vi "Multirecord Acquisition (FPGA) - original.vi"() -> ()   [LabVIEW 2021]
doc: "Use this VI as a template for the reconfigurable oscilloscope acquisition design. The block diagram is divided into three main loops.\n\nRegister Bus: This loop initializes the registers that are needed to support the configuration of the device. The FIFO bus, on the left, allows all the other design libraries to communicate with one another. This loop is very important to support the proper behavior of the instrument design library components.\n\nAcquisition: Acquires data from the I/O channels and writes the data into the record memory using the <B>Write</B> VI of the Multirecord Acquisition instrument design library. This VI also evaluates the various acquisition triggers and decides whether to acquire each data value in record memory. The host level VI (Fetch Record.vi) can read acquired records from the DRAM. The data is stored in 2 DRAM banks, each with 768 MB of storage.\n\nFetch: The recorded data is retrieved when the <B>Fetch Single Record</B> VI is run from the host VI. The <B>Write to Fetch DMA FIFO</B> VI writes data to the acq.fetch fifo 0 to transmit record data form the FPGA to the record fetch VIs on the host. This DMA FIFO must have a predefined name based on the instance parameter. By default, it is 0 (since the associated terminal on the <B>Create Resources DRAM Write Read</B> VI is unwired), so the connected FIFO is named acq.fetch fifo 0."
uses:
  Trigger/SubVIs/Types/Trigger Type.ctl
  <instrlib>/_niInstr/Data Trigger/v1/Shared/Public/Level Configuration FXP(+-,18,1).ctl
  <instrlib>/_niInstr/Data Trigger/v1/Shared/Public/Level Configuration Trigger When.ctl
  <instrlib>/_niInstr/Data Trigger/v1/Shared/Public/Edge Configuration FXP(+-,18,1).ctl
  <instrlib>/_niInstr/Data Trigger/v1/Shared/Public/Edge Configuration Trigger Slope.ctl
  FPGA Interface Typedefinitions/Trigger Combination Type.ctl
  <vilib>/Platform/TimedLoop/XDataNode/timing_clust.ctl
  <vilib>/Platform/TimedLoop/XDataNode/nitl_modes.ctl
  <vilib>/Platform/TimedLoop/XDataNode/wakeup.ctl
  <instrlib>/_niInstr/FIFO Register Bus/v1/FPGA/niInstr FIFO Register Bus v1 FPGA.lvclass
  C:/Program Files (x86)/National Instruments/LabVIEW 2021/instr.lib/_niInstr/Instruction Framework/v1/FPGA/Interfaces/Instruction Producer/Instruction Producer.lvclass
  <instrlib>/_niInstr/Multirecord Acquisition/Common/v1/FPGA/niInstr Multirecord Acquisition Common v1 FPGA.lvclass
  C:/Program Files (x86)/National Instruments/LabVIEW 2021/instr.lib/_niInstr/Multirecord Acquisition/Interface/v1/FPGA/niInstr Multirecord Acquisition v1 FPGA.lvclass
  <vilib>/rvi/Emulation/niFpgaSctlEmulationGetInTimedLoop.vi
  <vilib>/rvi/Emulation/niFpgaEmulationReportErrorSimple.vi
  <vilib>/rvi/Emulation/niFpgaGetClockAttributes.vi
  <vilib>/rvi/Emulation/niFpgaCriticalErrorInLSC.vi
  <instrlib>/_niInstr/Multirecord Acquisition/Common/v1/FPGA/Private/Create Fetch DMA FIFO Resources U8x32.vi
  <instrlib>/_niInstr/Multirecord Acquisition/Common/v1/FPGA/Private/Create Resources DRAM U384x2 U768 Write Read.vi
  <instrlib>/_niInstr/Multirecord Acquisition/Interface/v1/FPGA/Private/Retrieve Record U16 Wrapper.vi
  <instrlib>/_niInstr/Multirecord Acquisition/Interface/v1/FPGA/Private/Write to Fetch DMA FIFO U16 Wrapper.vi
  <vilib>/rvi/eio/common/nirviEmuTemplateMethod_errors.vi
  <instrlib>/HSAI-RIO/Config/Group A/v1/FPGA/Digital Correction/Validate 8 Channel Data.vi
  <instrlib>/HSAI-RIO/Config/Group A/v1/FPGA/Digital Correction/Digital Correction (8 Ch).vi
  <instrlib>/HSAI-RIO/Config/Group A/v1/FPGA/Digital Correction/FIR Filter (8 Ch).vi
  DSP/SubVIs/Integer decimationx8ch.vi
  Data Type Conversion/SubVIs/Remove Overflow FXP(+-,18,1)x8ch.vi
  <instrlib>/_niInstr/Channel/v1/FPGA/Private/Select/Select FXP(+-,18,1,)xNspcx8ch.vi
  Data Type Conversion/SubVIs/Data Type Conversion FXP(+-,18,1) to I16x8ch.vi
  <instrlib>/_niInstr/Channel/v1/FPGA/Private/Select and Interleave/Select And Interleave I16xNspcx8ch.vi
  Trigger/Trigger FXP(+,-,18,1).vi
  <instrlib>/_niInstr/Multirecord Acquisition/Interface/v1/FPGA/Private/Write I16 Wrapper.vi
  <vilib>/Platform/TimedLoop/XDataNode/XDataNode.xnode
  <vilib>/eio/EIONode/EIONode.xnode
  <instrlib>/_niInstr/Instruction Framework/v1/FPGA/Top Level Bus/Register Configuration/Register Configuration.lvclass
  <vilib>/Platform/TimedLoop/XDataNode/XDNodeRunTimeDep.lvlib
  <instrlib>/_niInstr/Multirecord Acquisition/Interface/v1/FPGA/niInstr Multirecord Acquisition v1 FPGA.lvclass
  <vilib>/rvi/LocalResourceManager/LocalResourceManager.xnode
  <vilib>/rvi/eio/common/nirviEmuReportErrorAndStop.vi
  <vilib>/rvi/DataTransferAndStorage/Container/Common/niFpgaContainerGetUniqueNameForEmu.vi
  <vilib>/rvi/DataTransferAndStorage/Container/Common/niFpgaContainerSetEmuInfo.vi
  <instrlib>/_niInstr/Channel/v1/FPGA/niInstr Channel v1 FPGA.lvlib
  <instrlib>/_niInstr/Basic Elements/v1/FPGA/niInstr Basic Elements v1 FPGA.lvlib
  <instrlib>/HSAI-RIO/Config/Group A/v1/FPGA/Digital Correction/Digital Correction.lvclass
  <instrlib>/HSAI-RIO/Config/Group A/v1/FPGA/Config Registers/Config Registers.lvclass
  <instrlib>/_niInstr/Data Trigger/v1/Shared/niInstr Data Trigger v1 Shared.lvlib
  <instrlib>/_niInstr/Multirecord Acquisition/Common/v1/FPGA/Private/Create Resources DRAM U384.vi
  <instrlib>/_niInstr/Multirecord Acquisition/Common/v1/FPGA/Private/Create Resources BRAM U384.vi
  Emulation/SubVIs/2 Element Generate Sine Cos Data FXP(+,-,14,1).vi
  <instrlib>/HSAI-RIO/Config/Group A/v1/FPGA/Digital Correction/Validate 4 Channel Data.vi
  <instrlib>/HSAI-RIO/Config/Group A/v1/FPGA/Digital Correction/Digital Correction (4 Ch).vi
  <instrlib>/_niInstr/Channel/v1/FPGA/Private/Select/Select FXP(+-,18,1,)xNspcx4ch.vi
  C:/Program Files (x86)/National Instruments/LabVIEW 2021/instr.lib/_niInstr/Multirecord Acquisition/Common/v1/FPGA/niInstr Multirecord Acquisition Common v1 FPGA.lvclass
  Data Type Conversion/SubVIs/Remove Overflow FXP(+-,18,1)x4ch.vi
  Data Type Conversion/SubVIs/Data Type Conversion FXP(+-,18,1) to I16x4ch.vi
  <instrlib>/_niInstr/Channel/v1/FPGA/Private/Select and Interleave/Select And Interleave I16xNspcx4ch.vi
  DSP/SubVIs/Integer decimationx4ch.vi
  <instrlib>/HSAI-RIO/Config/Group A/v1/FPGA/Digital Correction/FIR Filter (4 Ch).vi
  <instrlib>/_niInstr/Multirecord Acquisition/Common/v1/FPGA/Private/Create Resources BRAM U768.vi
  FPGA Interface Typedefinitions/FPGA Interface Typedefinitions.lvlib
panel:
  in  "trigger.rearm delay":u16=2
  in  "start trigger":bool=TRUE
  in  "trigger.type B":T1
  in  "reset":bool
  in  "trigger.combination type":T2
  in  "trigger.edge B":T3
  in  "trigger.level B":T5
  in  "trigger.edge A":T3
  in  "trigger.level A":T5
  in  "trigger.type A":T1
  in  "trigger.channel A":u8
  in  "trigger.channel B":u8
  out "fifo reg bus data 0":u64
  out "fifo reg bus status 0":u32
  in  "fifo reg bus ctrl 0":u32
  out "overflow":bool
  in  "dsp.decimation factor":u16
  out "overload":bool
  in  "channel.enable mask":u16=65535 format="%.0b"
  in  "channel.number of channels":u8=8
  # "Register Bus Controls"
  # "FPGA"
  # "Acquisition Loop Controls"
  # "DSP"
  # "Trigger"
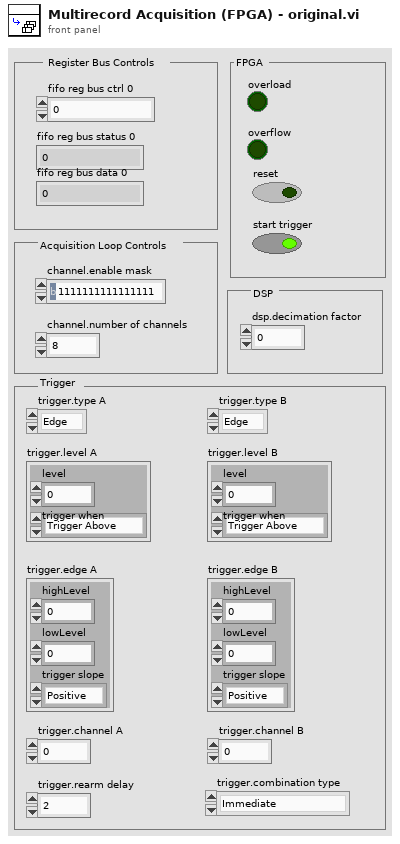
[diagram p1: front panel]
types:
  T1 = typedef "Trigger Type.ctl" = enum16{"Edge", "Level", "Custom"}
  T2 = typedef "FPGA Interface Typedefinitions.lvlib/Trigger Combination Type.ctl" = enum16{"Immediate", "A", "B", "OR", "AND", "A THEN B", "B THEN A", "High Resolution"}
  T3 = typedef "niInstr Data Trigger v1 Shared.lvlib/Edge Configuration FXP(+-,18,1).ctl" = cluster{"highLevel":fxp<+/-,18,1>, "lowLevel":fxp<+/-,18,1>, "trigger slope":T4}
  T4 = typedef "niInstr Data Trigger v1 Shared.lvlib/Edge Configuration Trigger Slope.ctl" = enum8{"Positive", "Negative"}
  T5 = typedef "niInstr Data Trigger v1 Shared.lvlib/Level Configuration FXP(+-,18,1).ctl" = cluster{"level":fxp<+/-,18,1>, "trigger when":T6}
  T6 = typedef "niInstr Data Trigger v1 Shared.lvlib/Level Configuration Trigger When.ctl" = enum8{"Trigger Above", "Trigger Below"}
  T7 = cluster{"memory 1":refnum<k21>, "memory 2":refnum<k21>}
  T8 = typedef "XDNodeRunTimeDep.lvlib/timing_clust.ctl" = cluster{"Expected End [f-1]":u64, "Actual End [f-1]":u64, "Finished Late? [f-1]":bool, "Expected End [i-1]":u64, "Actual End [i-1]":u64, "Finished Late? [i-1]":bool, "Expected Start [i]":u64, "Actual Start [i]":u64, "Expected Start [f]":u64, "Actual Start [f]":u64, "Source Name":string, "Structure Name":string, "Period":i64, "Deadline":i64, "Offset":i64, "Start":i64, "Priority":i32, "Timeout":i32, "Mode":T9, "Wakeup Reason":T10, "Error":errorcluster, "Source Type":string, "Secondary Source Type":string, "Global End Time":u64, "Global Start Time":u64, "Frame Duration":u64, "Iteration Duration":u64, "Assigned CPU":i32, "I/O Scan Engine Mode":u32}
  T9 = typedef "XDNodeRunTimeDep.lvlib/nitl_modes.ctl" = enum32{"No Change", "Process missed periods, maintain original phase", "Discard missed periods, maintain original phase", "Process missed periods, ignore original phase", "Discard missed periods, ignore original phase"}
  T10 = typedef "XDNodeRunTimeDep.lvlib/wakeup.ctl" = enum32{"Normal", "Aborted", "Asynchronous wakeup", "Timing source error", "Timed loop error", "Timeout"}
  T11 = typedef "niInstr Multirecord Acquisition v1 FPGA.lvclass/Timestamp.ctl" = cluster{"timestamp":u64, "valid":bool}
  T12 = typedef "niInstr Types v1 Shared.lvlib/Input Triggers.ctl" = cluster{"start":bool, "advance":bool, "reference":bool, "start trigger index":u16, "advance trigger index":u16, "reference trigger index":u16, "reference trigger correction cycle count":u32}
  T13 = cluster{"Channel 0":fxp<+/-,14,1>[], "Channel 1":fxp<+/-,14,1>[], "Channel 2":fxp<+/-,14,1>[], "Channel 3":fxp<+/-,14,1>[], "Channel 4":fxp<+/-,14,1>[], "Channel 5":fxp<+/-,14,1>[], "Channel 6":fxp<+/-,14,1>[], "Channel 7":fxp<+/-,14,1>[]}
  T14 = cluster{"Channel 0":fxp<+/-,18,1>[], "Channel 1":fxp<+/-,18,1>[], "Channel 2":fxp<+/-,18,1>[], "Channel 3":fxp<+/-,18,1>[], "Channel 4":fxp<+/-,18,1>[], "Channel 5":fxp<+/-,18,1>[], "Channel 6":fxp<+/-,18,1>[], "Channel 7":fxp<+/-,18,1>[]}
  T15 = cluster{"channel 0":fxp<+/-,18,1>[], "channel 1":fxp<+/-,18,1>[], "channel 2":fxp<+/-,18,1>[], "channel 3":fxp<+/-,18,1>[], "channel 4":fxp<+/-,18,1>[], "channel 5":fxp<+/-,18,1>[], "channel 6":fxp<+/-,18,1>[], "channel 7":fxp<+/-,18,1>[]}
  T16 = cluster{"channel 0":i16[], "channel 1":i16[], "channel 2":i16[], "channel 3":i16[], "channel 4":i16[], "channel 5":i16[], "channel 6":i16[], "channel 7":i16[]}
  T17 = typedef "niInstr Types v1 Shared.lvlib/Sample Format.ctl" = cluster{"bits per channel":u16, "samples per clock":u16, "channels":u8}
  T18 = cluster{"Channel 0":fxp<+/-,14,1>[], "Channel 1":fxp<+/-,14,1>[], "Channel 2":fxp<+/-,14,1>[], "Channel 3":fxp<+/-,14,1>[]}
  T19 = cluster{"Channel 0":fxp<+/-,18,1>[], "Channel 1":fxp<+/-,18,1>[], "Channel 2":fxp<+/-,18,1>[], "Channel 3":fxp<+/-,18,1>[]}
  T20 = cluster{"channel 0":fxp<+/-,18,1>[], "channel 1":fxp<+/-,18,1>[], "channel 2":fxp<+/-,18,1>[], "channel 3":fxp<+/-,18,1>[]}
  T21 = cluster{"channel 0":i16[], "channel 1":i16[], "channel 2":i16[], "channel 3":i16[]}
  T22 = typedef "niInstr Multirecord Acquisition v1 FPGA.lvclass/Events.ctl" = cluster{"ready for start":bool, "ready for advance":bool, "ready for reference":bool, "end of record":bool, "done":bool, "start trigger":bool, "advance trigger":bool, "reference trigger":bool, "start trigger index":u16, "advance trigger index":u16, "reference trigger index":u16}
  T23 = typedef "niInstr Multirecord Acquisition v1 FPGA.lvclass/Retrieve Data Info.ctl" = cluster{"read request size (bits)":u64, "valid data offset (bits)":u16, "valid data size (bits)":u16, "first sample of request":bool, "last sample of request":bool, "Token":T24}
  T24 = typedef "niInstr Types v1 Shared.lvlib/Token.ctl" = cluster{"identifier":u8, "value":u32}
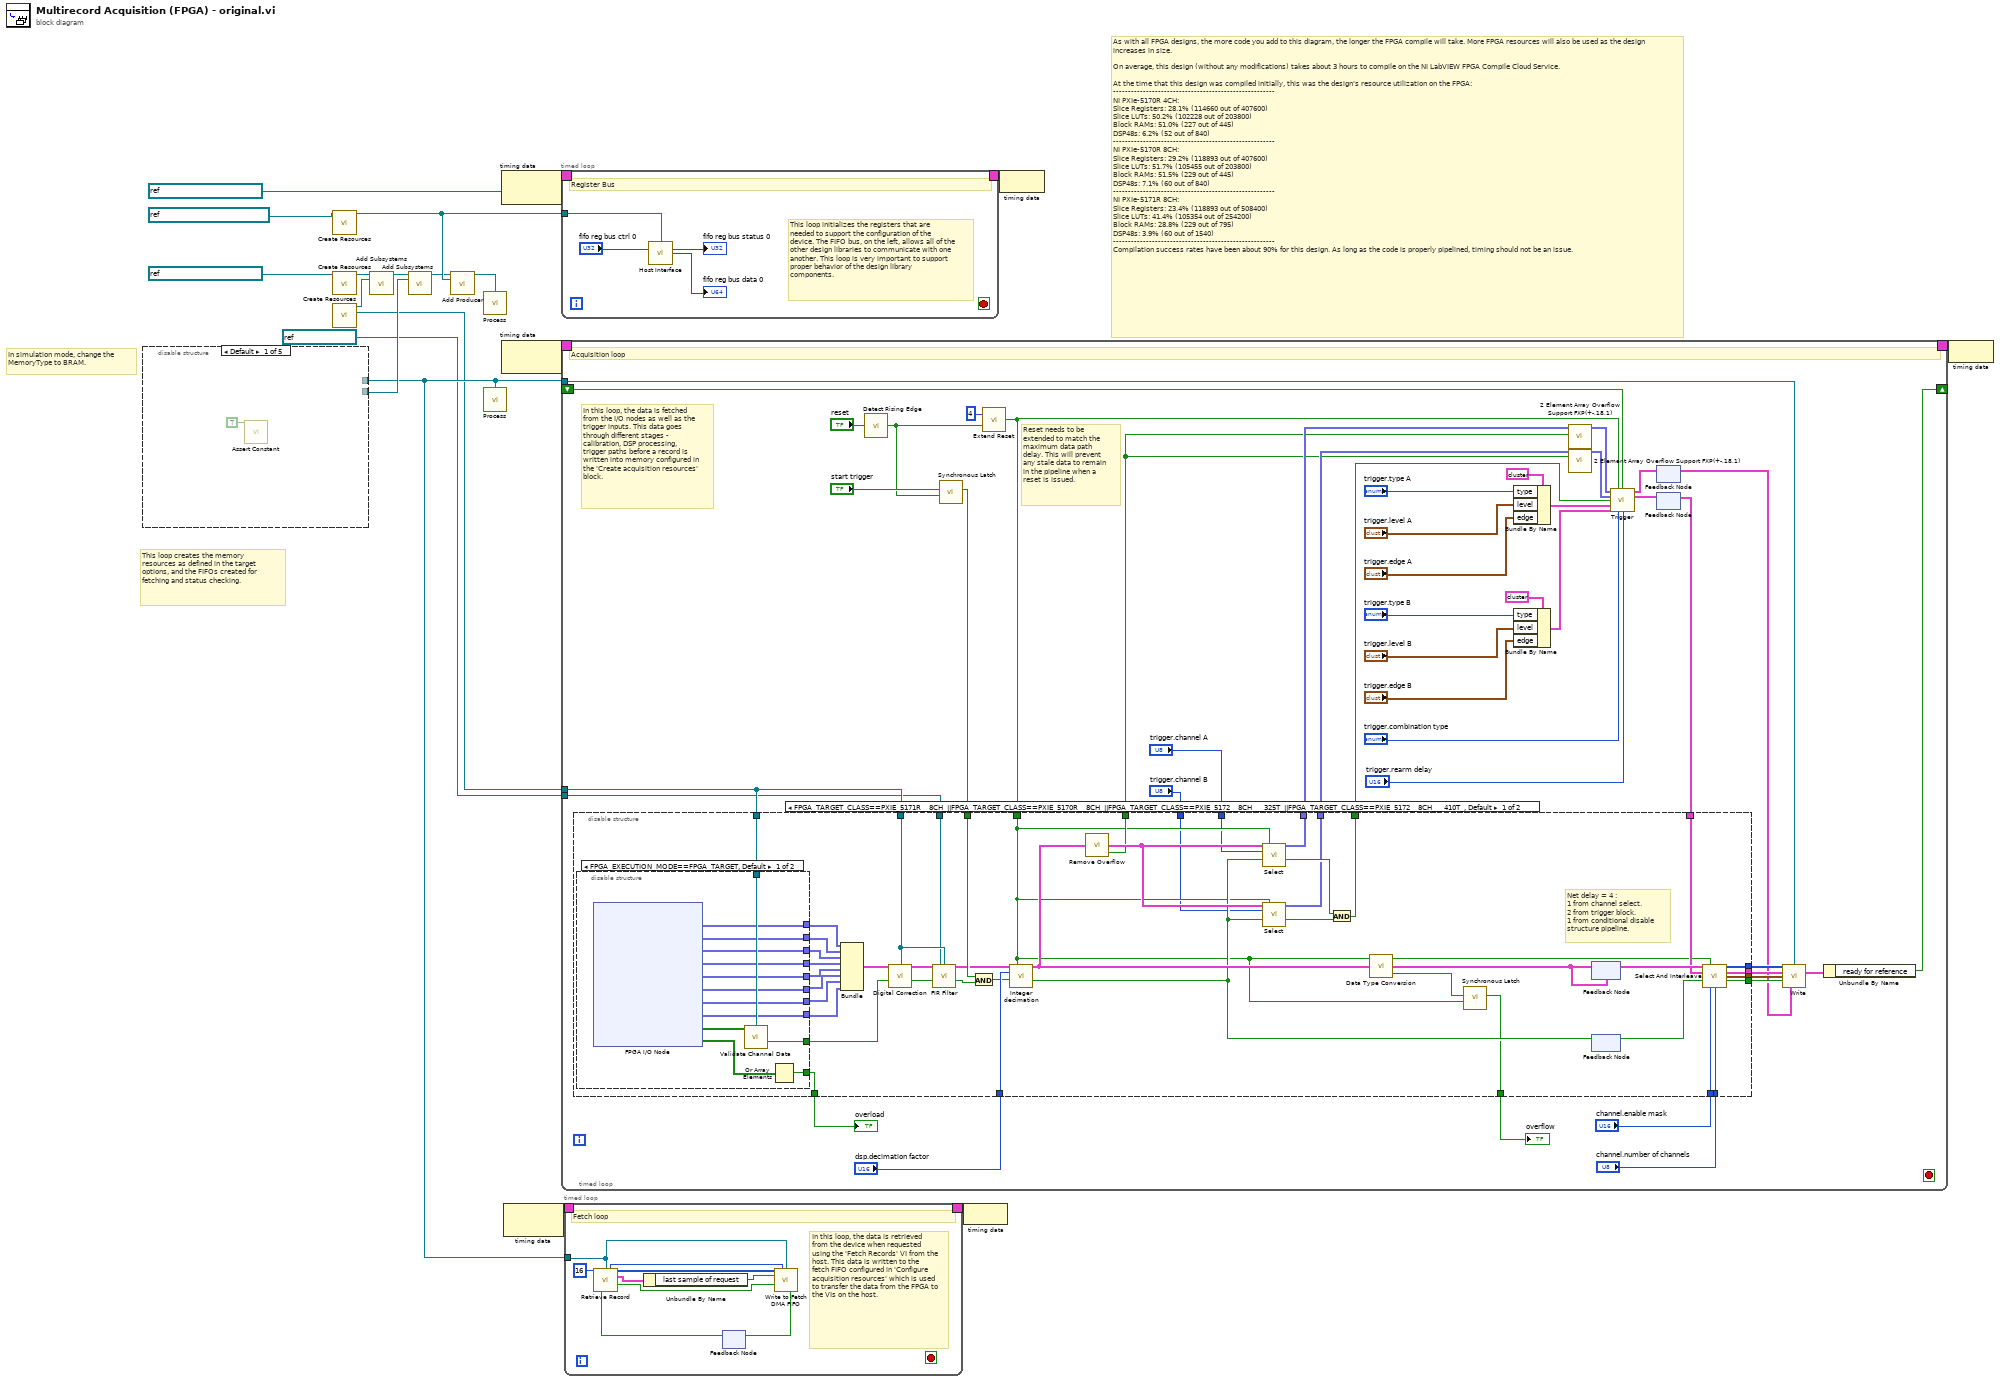
[diagram p0: block diagram]
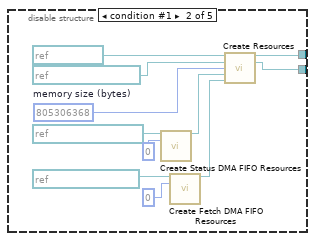
[diagram p2: hidden frame]
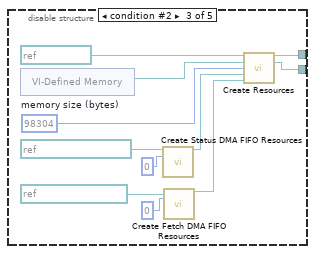
[diagram p3: hidden frame]
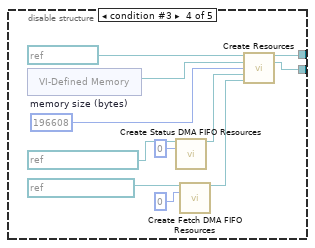
[diagram p4: hidden frame]
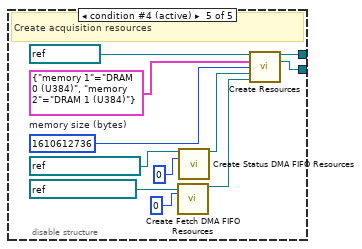
[diagram p5: hidden frame]
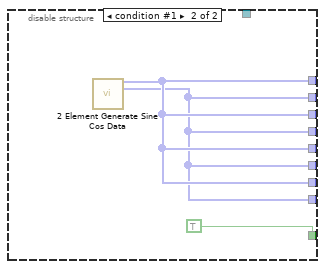
[diagram p6: hidden frame]
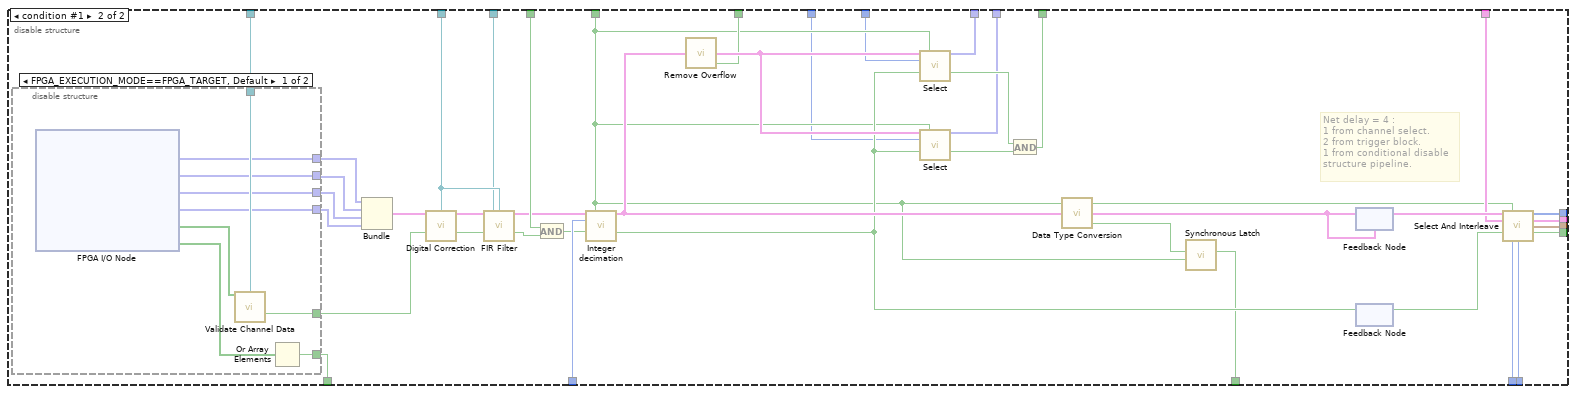
[diagram p7: hidden frame]
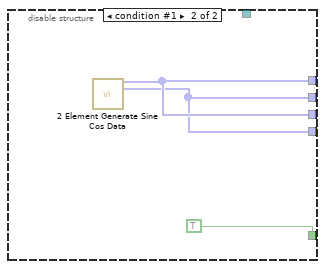
[diagram p8: hidden frame]
diagram:
  # "In simulation mode, change the MemoryType to BRAM."
  # "This loop creates the memory resources as defined in the target options, and the FIFOs created for fetching and status checking."
  # "As with all FPGA designs, the more code you add to this diagram, the longer the FPGA compile will take. More FPGA resources will also be used as the design increases in size.\n\nOn average, this design (without any modifications) takes about 3 hours to compile on the NI LabVIEW FPGA Compile Cloud Service. \n\nAt the time that this design was compiled initially, this was the design's resource utilization on the FPGA:\n------------------------------------------------------\nNI PXIe-5170R 4CH:\nSlice Registers: 28.1% (114660 out of 407600)\nSlice LUTs: 50.2% (102228 out of 203800)\nBlock RAMs: 51.0% (227 out of 445)\nDSP48s: 6.2% (52 out of 840)\n------------------------------------------------------\nNI PXIe-5170R 8CH:\nSlice Registers: 29.2% (118893 out of 407600)\nSlice LUTs: 51.7% (105455 out of 203800)\nBlock RAMs: 51.5% (229 out of 445)\nDSP48s: 7.1% (60 out of 840)\n------------------------------------------------------\nNI PXIe-5171R 8CH:\nSlice Registers: 23.4% (118893 out of 508400)\nSlice LUTs: 41.4% (105354 out of 254200)\nBlock RAMs: 28.8% (229 out of 795)\nDSP48s: 3.9% (60 out of 1540)\n------------------------------------------------------\nCompilation success rates have been about 90% for this design. As long as the code is properly pipelined, timing should not be an issue."
  n1 = disable-structure shown="Default" {
    disable-tunnel: [_ w29 w40 w51 w62] -> w4
    disable-tunnel: [_ w26 w36 w47 w59] -> w7
    frame condition #0 {
      n2 = call <instrlib>:"Assert Constant.vi"("constant terminal"=TRUE) -> ()  [unwired: 15 in]
    }
    frame condition #1 {
      w30 = u64 805306368  # memory size (bytes)
      n3 = call <instrlib>:"Create Status DMA FIFO Resources.vi"("status dma fifo in"=refnum<k21> "acq.status fifo 0" ("status dma fifo"), "fifo instance"=u8 0) -> ("status dma fifo out"=w21:refnum<class "niInstr Status FIFO v1 FPGA.lvclass">)  [unwired: 13 in]
      n4 = call-poly <instrlib>:"Create Fetch DMA FIFO Resources.vi"("fetch dma fifo in"=refnum<k21> "acq.fetch fifo 0", "fifo instance"=u8 0) -> ("fetch dma fifo out"=w27:refnum<class "niInstr Fetch FIFO v1 FPGA.lvclass">)  [unwired: 13 in]
      n5 = call-poly <instrlib>:"Create Resources.vi"("memory clock"=refnum<k21> "160MHz" ("process clock"), "memory"=refnum<k21> "DRAM 0 (U384)" ("dram"), "memory size (bytes)"=w30, "status dma fifo resources"=w21, "fetch dma fifo resources"=w27) -> ("acquisition resources"=w29:refnum<class "niInstr Multirecord Acquisition Common v1 FPGA.lvclass">, "acquisition subsystem"=w26:refnum<class "Address Space Collection.lvclass">)  [unwired: 9 in]
    }
    frame condition #2 {
      w41 = u64 98304  # memory size (bytes)
      n6 = xnode "VI-Defined Memory"() -> ("Memory Out"=w42:refnum<k21>)
      n7 = call <instrlib>:"Create Status DMA FIFO Resources.vi"("status dma fifo in"=refnum<k21> "acq.status fifo 0" ("status dma fifo"), "fifo instance"=u8 0) -> ("status dma fifo out"=w33:refnum<class "niInstr Status FIFO v1 FPGA.lvclass">)  [unwired: 13 in]
      n8 = call-poly <instrlib>:"Create Fetch DMA FIFO Resources.vi"("fetch dma fifo in"=refnum<k21> "acq.fetch fifo 0", "fifo instance"=u8 0) -> ("fetch dma fifo out"=w37:refnum<class "niInstr Fetch FIFO v1 FPGA.lvclass">)  [unwired: 13 in]
      n9 = call-poly <instrlib>:"Create Resources.vi"("memory clock"=refnum<k21> "160MHz" ("process clock"), "memory"=w42, "memory size (bytes)"=w41, "status dma fifo resources"=w33, "fetch dma fifo resources"=w37) -> ("acquisition resources"=w40:refnum<class "niInstr Multirecord Acquisition Common v1 FPGA.lvclass">, "acquisition subsystem"=w36:refnum<class "Address Space Collection.lvclass">)  [unwired: 9 in]
    }
    frame condition #3 {
      w52 = u64 196608  # memory size (bytes)
      n10 = xnode "VI-Defined Memory"() -> ("Memory Out"=w53:refnum<k21>)
      n11 = call <instrlib>:"Create Status DMA FIFO Resources.vi"("status dma fifo in"=refnum<k21> "acq.status fifo 0" ("status dma fifo"), "fifo instance"=u8 0) -> ("status dma fifo out"=w45:refnum<class "niInstr Status FIFO v1 FPGA.lvclass">)  [unwired: 13 in]
      n12 = call-poly <instrlib>:"Create Fetch DMA FIFO Resources.vi"("fetch dma fifo in"=refnum<k21> "acq.fetch fifo 0", "fifo instance"=u8 0) -> ("fetch dma fifo out"=w48:refnum<class "niInstr Fetch FIFO v1 FPGA.lvclass">)  [unwired: 13 in]
      n13 = call-poly <instrlib>:"Create Resources.vi"("memory clock"=refnum<k21> "160MHz" ("process clock"), "memory"=w53, "memory size (bytes)"=w52, "status dma fifo resources"=w45, "fetch dma fifo resources"=w48) -> ("acquisition resources"=w51:refnum<class "niInstr Multirecord Acquisition Common v1 FPGA.lvclass">, "acquisition subsystem"=w47:refnum<class "Address Space Collection.lvclass">)  [unwired: 9 in]
    }
    frame condition #4 (active) {
      w64 = u64 1610612736  # memory size (bytes)
      # "Create acquisition resources"
      n14 = call-poly <instrlib>:"Create Fetch DMA FIFO Resources.vi"("fetch dma fifo in"=refnum<k21> "acq.fetch fifo 0", "fifo instance"=u8 0) -> ("fetch dma fifo out"=w61:refnum<class "niInstr Fetch FIFO v1 FPGA.lvclass">)  [unwired: 13 in]
      n15 = call <instrlib>:"Create Status DMA FIFO Resources.vi"("status dma fifo in"=refnum<k21> "acq.status fifo 0" ("status dma fifo"), "fifo instance"=u8 0) -> ("status dma fifo out"=w56:refnum<class "niInstr Status FIFO v1 FPGA.lvclass">)  [unwired: 13 in]
      n16 = call-poly <instrlib>:"Create Resources.vi"("memory clock"=refnum<k21> "160MHz" ("process clock"), "memory"=T7 {"memory 1"="DRAM 0 (U384)", "memory 2"="DRAM 1 (U384)"}, "memory size (bytes)"=w64, "status dma fifo resources"=w56, "fetch dma fifo resources"=w61) -> ("acquisition resources"=w62:refnum<class "niInstr Multirecord Acquisition Common v1 FPGA.lvclass">, "acquisition subsystem"=w59:refnum<class "Address Space Collection.lvclass">)  [unwired: 9 in]
    }
  }
  n17 = call <instrlib>:"Create Resources.vi"("instruction fifo"=refnum<k21> "reg.host instruction fifo 0" ("FIFO")) -> ("fifo register bus"=w6:refnum<class "niInstr FIFO Register Bus v1 FPGA.lvclass">)  [unwired: 14 in]
  n18 = call <instrlib>:"Create Resources.vi"("register clock"=refnum<k21> "40 MHz Onboard Clock" ("Source Name")) -> ("register configuration"=w10:refnum<class "Register Configuration.lvclass">)  [unwired: 14 in]
  n19 = call <instrlib>:"Create Resources.vi"() -> ("config subsystems"=w8:refnum<class "Address Space Collection.lvclass">, "digital correction resources"=w1:refnum<class "Digital Correction.lvclass">)  [unwired: 14 in]
  n20 = call-dynamic "Add Subsystems.vi"("register configuration in"=w10, "subsystems"=w8) -> ("register configuration out"=w9:refnum<class "Register Configuration.lvclass">)  [unwired: 13 in]
  n21 = call-dynamic "Add Subsystems.vi"("register configuration in"=w9, "subsystems"=w7) -> ("register configuration out"=w3:refnum<class "Register Configuration.lvclass">)  [unwired: 13 in]
  n22 = call-dynamic "Add Producer.vi"("register configuration in"=w3, "instruction producer"=w6) -> ("register configuration out"=w5:refnum<class "Register Configuration.lvclass">)  [unwired: 13 in]
  n23 = call-dynamic "Process.vi"("register configuration"=w5) -> ()  [unwired: 15 in]
  n24 = call-dynamic "Process.vi"("acquisition resources"=w4) -> ()  [unwired: 15 in]
  n25 = node-c288(refnum<k21> "40 MHz Onboard Clock" ("Source Name")) -> (w19:T8)
  n26 = node-c288() -> (w17:T8)  [unwired: 1 in]
  n27 = node-c288() -> (w15:T8)  [unwired: 1 in]
  n28 = timed-loop {
    timing: w19 -> [_]
    timing-out: [_] -> w18
    tunnel: w6 -> [w68]
    stop <- _ stop-if-true
    # "This loop initializes the registers that are needed to support the configuration of the device. The FIFO bus, on the left, allows all of the other design libraries to communicate with one another. This loop is very important to support proper behavior of the design library components."
    # "Register Bus"
    n29 = call <instrlib>:"Host Interface.vi"("fifo register bus"=w68, "fifo reg bus ctrl 0"="fifo reg bus ctrl 0") -> ("fifo reg bus status 0"=→"fifo reg bus status 0":u32, "fifo reg bus data 0"=→"fifo reg bus data 0":u64)  [unwired: 12 in]
  }
  n30 = timed-loop {
    timing: w17 -> [_]
    timing-out: [_] -> w16
    tunnel: w4 -> [w114]
    tunnel: w1 -> [w76]
    shift-right: [w105] -> _
    shift-left: _ -> [w100]
    tunnel: refnum<k21> "Data Clock x2" -> [w71]
    stop <- _ stop-if-true
    # "Reset needs to be extended to match the maximum data path delay. This will prevent any stale data to remain in the pipeline when a reset is issued."
    # "In this loop, the data is fetched from the I/O nodes as well as the trigger inputs. This data goes through different stages - calibration, DSP processing, trigger paths before a record is written into memory configured in the 'Create acquisition resources' block."
    # "Acquisition loop"
    n31 = call <instrlib>:"Detect Rising Edge.vi"("signal"="reset") -> ("edge detected"=w73:bool)  [unwired: 14 in]
    n32 = call <instrlib>:"Synchronous Latch.vi"("clear"=w73, "set"="start trigger") -> ("out"=w84:bool)  [unwired: 9 in]
    n33 = call "Extend Reset.vi"("reset in"=w73, "number of cycles"=u8 4) -> ("reset out"=w74:bool)
    n34 = Bundle By Name(cluster=cluster{"type":T1, "level":T5, "edge":T3} {"type"=enum."Edge", "level"={"level"=0.0, "trigger when"=enum."Trigger Above"}, "edge"={"highLevel"=0.0, "lowLevel"=0.0, "trigger slope"=enum."Positive"}} ("trigger.A"), "type"="trigger.type A", "level"="trigger.level A", "edge"="trigger.edge A") -> (w94:cluster{"type":T1, "level":T5, "edge":T3})
    n35 = Bundle By Name(cluster=cluster{"type":T1, "level":T5, "edge":T3} {"type"=enum."Edge", "level"={"level"=0.0, "trigger when"=enum."Trigger Above"}, "edge"={"highLevel"=0.0, "lowLevel"=0.0, "trigger slope"=enum."Positive"}} ("trigger.A"), "type"="trigger.type B", "level"="trigger.level B", "edge"="trigger.edge B") -> (w93:cluster{"type":T1, "level":T5, "edge":T3})
    n36 = feedback #1() -> (w80:T11)  [unwired: 1 in]
    n37 = feedback #2() -> (w82:T12)  [unwired: 1 in]
    n38 = disable-structure shown="FPGA_TARGET_CLASS==PXIE_5171R__8CH_||FPGA_TARGET_CLASS==PXIE_5170R__8CH_||FPGA_TARGET_CLASS==PXIE_5172__8CH___325T_||FPGA_TARGET_CLASS==PXIE_5172__8CH___410T_, Default" {
      disable-tunnel: w76 -> [w118 w179]
      disable-tunnel: "channel.number of channels" -> [w159 w215]
      disable-tunnel: [w150 w210] -> w113
      disable-tunnel: [w149 w209] -> w112
      disable-tunnel: [w148 w208] -> w111
      disable-tunnel: [w147 w207] -> w110
      disable-tunnel: [w146 w206] -> w109
      disable-tunnel: "dsp.decimation factor" -> [w145 w205]
      disable-tunnel: "channel.enable mask" -> [w142 w202]
      disable-tunnel: w82 -> [w139 w199]
      disable-tunnel: [w137 w197] -> w92
      disable-tunnel: [w134 w194] -> w90
      disable-tunnel: [w133 w193] -> w88
      disable-tunnel: [w128 w188] -> w86
      disable-tunnel: w84 -> [w126 w186]
      disable-tunnel: w74 -> [w125 w185]
      disable-tunnel: "trigger.channel A" -> [w124 w184]
      disable-tunnel: "trigger.channel B" -> [w123 w183]
      disable-tunnel: [w122 w182] -> w77
      disable-tunnel: w76 -> [_ _]
      disable-tunnel: w71 -> [w117 w178]
      frame condition #0 (active) {
        # "Net delay = 4 :\n1 from channel select.\n2 from trigger block.\n1 from conditional disable structure pipeline."
        n39 = disable-structure shown="FPGA_EXECUTION_MODE==FPGA_TARGET, Default" {
          disable-tunnel: [w170 w175] -> w158
          disable-tunnel: [w169 w174] -> w157
          disable-tunnel: [w168 w175] -> w156
          disable-tunnel: [w167 w174] -> w155
          disable-tunnel: [w166 w175] -> w154
          disable-tunnel: [w165 w174] -> w153
          disable-tunnel: [w164 w175] -> w151
          disable-tunnel: [w163 w174] -> w152
          disable-tunnel: [w160 TRUE ("ADC Data Valid")] -> w143
          disable-tunnel: w118 -> [w171 _]
          disable-tunnel: [w161 _] -> w150
          frame condition #0 (active) {
            # "I/O Nodes"
            n40 = xnode "FPGA I/O Node"() -> ("Channel 0"=w170:fxp<+/-,14,1>[], "Channel 1"=w169:fxp<+/-,14,1>[], "Channel 2"=w168:fxp<+/-,14,1>[], "Channel 3"=w167:fxp<+/-,14,1>[], "Channel 4"=w166:fxp<+/-,14,1>[], "Channel 5"=w165:fxp<+/-,14,1>[], "Channel 6"=w164:fxp<+/-,14,1>[], "Channel 7"=w163:fxp<+/-,14,1>[], "Channel Data Valid"=w172:bool[], "Channel Overload"=w162:bool[])  [unwired: 10 in, 10 out]
            n41 = call-poly <instrlib>:"Validate Channel Data.vi"("channel data valid"=w172, "digital correction resources"=w171) -> ("expected data valid"=w160:bool)  [unwired: 13 in]
            n42 = Or Array Elements(Boolean array=w162) -> (logical OR=w161:bool)
          }
          frame condition #1 {
            n43 = call-poly "2 Element Generate Sine Cos Data.vi"() -> ("sine data"=w175:fxp<+/-,14,1>[], "cosine data"=w174:fxp<+/-,14,1>[])  [unwired: 14 in]
          }
        }
        n44 = Bundle("Channel 0"=w158, "Channel 1"=w157, "Channel 2"=w156, "Channel 3"=w155, "Channel 4"=w154, "Channel 5"=w153, "Channel 6"=w151, "Channel 7"=w152) -> (w144:T13)  [unwired: 1 in]
        n45 = call-poly <instrlib>:"Digital Correction.vi"("channel data in"=w144, "digital correction resources"=w118, "input valid"=w143) -> ("corrected channel data out"=w121:T14, "output valid"=w120:bool)  [unwired: 11 in]
        n46 = call-poly <instrlib>:"FIR Filter.vi"("data in"=w121, "data clock x2"=w117, "digital correction resources"=w118, "input valid"=w120) -> ("data out"=w116:T14, "output valid"=w119:bool)  [unwired: 9 in, 1 out]
        n47 = And(x=w126, y=w119) -> (x .and. y?=w127:bool)
        n48 = call-poly "Integer decimation.vi"("data in"=w116, "reset"=w125, "decimation factor"=w145, "input valid"=w127) -> ("data out"=w132:T15, "output valid"=w130:bool)  [unwired: 9 in, 1 out]
        n49 = call-poly "Remove Overflow.vi"("data in"=w132) -> ("overflow"=w128:bool, "data out"=w138:T15)  [unwired: 3 in]
        n50 = call-poly <instrlib>:"Select.vi"("data in"=w138, "reset"=w125, "channel index"=w124, "input valid"=w130) -> ("channel out"=w134:fxp<+/-,18,1>[], "output valid"=w135:bool)  [unwired: 10 in]
        n51 = call-poly <instrlib>:"Select.vi"("data in"=w138, "reset"=w125, "channel index"=w123, "input valid"=w130) -> ("channel out"=w133:fxp<+/-,18,1>[], "output valid"=w136:bool)  [unwired: 10 in]
        n52 = And(x=w135, y=w136) -> (x .and. y?=w137:bool)
        n53 = call-poly "Data Type Conversion.vi"("data in"=w132) -> ("overflow"=w141:bool, "data out"=w131:T16)  [unwired: 3 in]
        n54 = call <instrlib>:"Synchronous Latch.vi"("clear"=w125, "set"=w141) -> ("out"=w122:bool)  [unwired: 9 in]
        n55 = feedback #3(w131) -> (w140:T16)
        n56 = feedback-in #3(w131) -> ()
        n57 = feedback #4() -> (w129:bool)  [unwired: 1 in]
        n58 = feedback-in #4(w130) -> ()
        n59 = call-poly <instrlib>:"Select And Interleave.vi"("data in"=w140, "reset"=w125, "triggers in"=w139, "input valid"=w129, "channel enable mask"=w142, "number of channels to interleave"=w159) -> ("interleaved data out"=w149:i16[], "triggers out"=w148:T12, "sample format out"=w147:T17, "output valid"=w146:bool)  [unwired: 5 in, 1 out]
      }
      frame condition #1 {
        # "Net delay = 4 :\n1 from channel select.\n2 from trigger block.\n1 from conditional disable structure pipeline."
        n60 = disable-structure shown="FPGA_EXECUTION_MODE==FPGA_TARGET, Default" {
          disable-tunnel: [w223 w227] -> w214
          disable-tunnel: [w222 w226] -> w213
          disable-tunnel: [w221 w227] -> w212
          disable-tunnel: [w220 w226] -> w211
          disable-tunnel: [w218 TRUE ("ADC Data Valid")] -> w203
          disable-tunnel: w179 -> [w224 _]
          disable-tunnel: [w219 _] -> w210
          frame condition #0 (active) {
            # "I/O Nodes"
            n61 = xnode "FPGA I/O Node"() -> ("Channel 0"=w223:fxp<+/-,14,1>[], "Channel 1"=w222:fxp<+/-,14,1>[], "Channel 2"=w221:fxp<+/-,14,1>[], "Channel 3"=w220:fxp<+/-,14,1>[], "Channel Data Valid"=w216:bool[], "Channel Overload"=w217:bool[])  [unwired: 6 in, 6 out]
            n62 = call-poly <instrlib>:"Validate Channel Data.vi"("channel data valid"=w216, "digital correction resources"=w224) -> ("expected data valid"=w218:bool)  [unwired: 13 in]
            n63 = Or Array Elements(Boolean array=w217) -> (logical OR=w219:bool)
          }
          frame condition #1 {
            n64 = call-poly "2 Element Generate Sine Cos Data.vi"() -> ("sine data"=w227:fxp<+/-,14,1>[], "cosine data"=w226:fxp<+/-,14,1>[])  [unwired: 14 in]
          }
        }
        n65 = Bundle("Channel 0"=w214, "Channel 1"=w213, "Channel 2"=w212, "Channel 3"=w211) -> (w204:T18)  [unwired: 1 in]
        n66 = call-poly <instrlib>:"Digital Correction.vi"("channel data in"=w204, "digital correction resources"=w179, "input valid"=w203) -> ("corrected channel data out"=w180:T19, "output valid"=w181:bool)  [unwired: 11 in]
        n67 = call-poly <instrlib>:"FIR Filter.vi"("data in"=w180, "data clock x2"=w178, "digital correction resources"=w179, "input valid"=w181) -> ("data out"=w177:T19, "output valid"=w176:bool)  [unwired: 9 in, 1 out]
        n68 = And(x=w186, y=w176) -> (x .and. y?=w187:bool)
        n69 = call-poly "Integer decimation.vi"("data in"=w177, "reset"=w185, "decimation factor"=w205, "input valid"=w187) -> ("data out"=w192:T20, "output valid"=w190:bool)  [unwired: 9 in, 1 out]
        n70 = call-poly "Remove Overflow.vi"("data in"=w192) -> ("overflow"=w188:bool, "data out"=w198:T20)  [unwired: 3 in]
        n71 = call-poly <instrlib>:"Select.vi"("data in"=w198, "reset"=w185, "channel index"=w184, "input valid"=w190) -> ("channel out"=w194:fxp<+/-,18,1>[], "output valid"=w195:bool)  [unwired: 10 in]
        n72 = call-poly <instrlib>:"Select.vi"("data in"=w198, "reset"=w185, "channel index"=w183, "input valid"=w190) -> ("channel out"=w193:fxp<+/-,18,1>[], "output valid"=w196:bool)  [unwired: 10 in]
        n73 = And(x=w195, y=w196) -> (x .and. y?=w197:bool)
        n74 = call-poly "Data Type Conversion.vi"("data in"=w192) -> ("overflow"=w201:bool, "data out"=w191:T21)  [unwired: 3 in]
        n75 = call <instrlib>:"Synchronous Latch.vi"("clear"=w185, "set"=w201) -> ("out"=w182:bool)  [unwired: 9 in]
        n76 = feedback #5(w191) -> (w200:T21)
        n77 = feedback-in #5(w191) -> ()
        n78 = feedback #6() -> (w189:bool)  [unwired: 1 in]
        n79 = feedback-in #6(w190) -> ()
        n80 = call-poly <instrlib>:"Select And Interleave.vi"("data in"=w200, "reset"=w185, "triggers in"=w199, "input valid"=w189, "channel enable mask"=w202, "number of channels to interleave"=w215) -> ("interleaved data out"=w209:i16[], "triggers out"=w208:T12, "sample format out"=w207:T17, "output valid"=w206:bool)  [unwired: 5 in, 1 out]
      }
    }
    "overload" <- w113
    "overflow" <- w77
    n81 = call "2 Element Array Overflow Support FXP(+-,18,1).vi"("data in"=w90, "overflow"=w86) -> ("data out"=w89:fxp<+/-,18,1>[])  [unwired: 13 in]
    n82 = call "2 Element Array Overflow Support FXP(+-,18,1).vi"("data in"=w88, "overflow"=w86) -> ("data out"=w87:fxp<+/-,18,1>[])  [unwired: 13 in]
    n83 = call-poly "Trigger.vi"("data A"=w89, "reset"=w74, "trigger.ready for reference"=w100, "data B"=w87, "input valid"=w92, "trigger.A"=w94, "trigger.B"=w93, "trigger.combination type"="trigger.combination type", "rearm delay"="trigger.rearm delay") -> ("timestamps"=w81:T11, "trigger.out"=w83:T12)  [unwired: 4 in, 1 out]
    n84 = feedback-in #1(w81) -> ()
    n85 = feedback-in #2(w83) -> ()
    n86 = call-poly <instrlib>:"Write.vi"("data"=w112, "acquisition resources"=w114, "triggers"=w111, "sample format"=w110, "data valid"=w109, "timestamp"=w80) -> ("events"=w106:T22)  [unwired: 7 in, 2 out]
    n87 = Unbundle By Name(w106) -> ("ready for reference"=w105:bool)
  }
  n88 = timed-loop {
    timing: w15 -> [_]
    timing-out: [_] -> w14
    tunnel: w4 -> [w238]
    stop <- _ stop-if-true
    # "In this loop, the data is retrieved from the device when requested using the 'Fetch Records' VI from the host. This data is written to the fetch FIFO configured in 'Configure acquisition resources' which is used to transfer the data from the FPGA to the VIs on the host."
    # "Fetch loop"
    n89 = feedback #7() -> (w236:bool)  [unwired: 1 in]
    n90 = call-poly <instrlib>:"Retrieve Record.vi"("output array size"=u16 16, "acquisition resources"=w238, "ready for output"=w236) -> ("channels"=w231:u8, "data"=w234:u16[], "retrieve data info"=w233:T23, "output valid"=w235:bool)  [unwired: 9 in]
    n91 = Unbundle By Name(w233) -> ("last sample of request"=w232:bool)
    n92 = call-poly <instrlib>:"Write to Fetch DMA FIFO.vi"("data"=w234, "channels"=w231, "acquisition resources"=w238, "last sample of request"=w232, "input valid"=w235) -> ("ready for input"=w237:bool)  [unwired: 10 in]
    n93 = feedback-in #7(w237) -> ()
  }
  n94 = node-c288(w14) -> ()
  n95 = node-c288(w18) -> ()
  n96 = node-c288(w16) -> ()
